vi "fpga_LP1 Process (M Class).vi"(0 "input data":fxp<+/-,32,3>, 1 "reset":bool, 2 "filter delay constant":T1, 5 "Ch":fxp<+,5,5>=6.0, 9 "input valid":bool, 12 "ready for output":bool) -> (4 "re":fxp<+/-,32,5> format="%.29g", 6 "im":fxp<+/-,32,5> format="%.29g", 10 "output valid":bool, 14 "ready for input":bool)   [LabVIEW 2013, in "NI_EP_PMU_FPGA.lvlib"]
uses:
  <vilib>/addons/Electrical Power/PMU/NI_EP_PMU_FPGA.lvlib
  <vilib>/addons/Electrical Power/PMU/FPGA/subVIs/fpga_Reporting Rate Configuration.ctl
  <vilib>/rvi/Emulation/niFpgaSctlEmulationGetInTimedLoop.vi
  <vilib>/rvi/DataTransferAndStorage/Container/Common/niFpgaContainerGetUniqueNameForEmu.vi
  <vilib>/rvi/DataTransferAndStorage/Container/Common/niFpgaContainerSetEmuInfo.vi
  <vilib>/rvi/eio/common/nirviEmuReportErrorAndStop.vi
  <vilib>/rvi/FIFO/Fifo_Resource/nirvififoEmulationSetSize.vi
  <vilib>/rvi/Emulation/niFpgaSctlEmulationFifoFullMgr.vi
  <vilib>/rvi/errors/niFpgaSetErrorForExecOnDevCompSimple.vi
  <vilib>/rvi/Memory/Memory_Emulation/nirvimemoryEmulation.vi
  <vilib>/rvi/Memory/Memory_Emulation/nirvimemoryFastEmulation.vi
  <vilib>/rvi/Memory/Memory_Emulation/niFpgaMemoryEmulationCacheClearOnFirstRun.vi
  <vilib>/rvi/Memory/Memory_Emulation/nirvimemoryEmulationManagerCache_MakeExclusive.vi
  <vilib>/rvi/Memory/Memory_Emulation/niFpgaMemoryEmulationValidateCache.vi
  <vilib>/rvi/Memory/Memory_Emulation/nirvimemoryEmulationManagerCache_ReleaseExclusive.vi
  <vilib>/rvi/Memory/Memory_Emulation/nirvimemoryEmulationManagerCache_InsertValue.vi
  <vilib>/Utility/error.llb/Clear Errors.vi
  <vilib>/rvi/Memory/Memory_Emulation/nirvimemoryEmulationManagerCache_GetValue.vi
  <vilib>/rvi/Emulation/niFpgaSctlEmulationResourceMgr.vi
  <vilib>/rvi/LocalResourceManager/LocalResourceManager.xnode
  <vilib>/rvi/DataTransferAndStorage/Container/XNode/niFpgaContainer.xnode
  <vilib>/rvi/FIFO/Fifo_Resource/nirvififoEmulationRead.vi
  <vilib>/rvi/FXPMathLib/basic elements/FxpDiscreteDelay/XNode/nifxpmath_DiscreteDelay.xnode
  <vilib>/rvi/FXPMathLib/FxpMul/XNode/nifxpmath_Multiplier.xnode
  <vilib>/rvi/FIFO/Fifo_Resource/nirvififoEmulationWrite.vi
  <vilib>/addons/Electrical Power/PQ/Resampling/NI_EP_Resample_FPGA.lvlib
  <vilib>/rvi/FXPMathLib/sim/FxpSim.dll
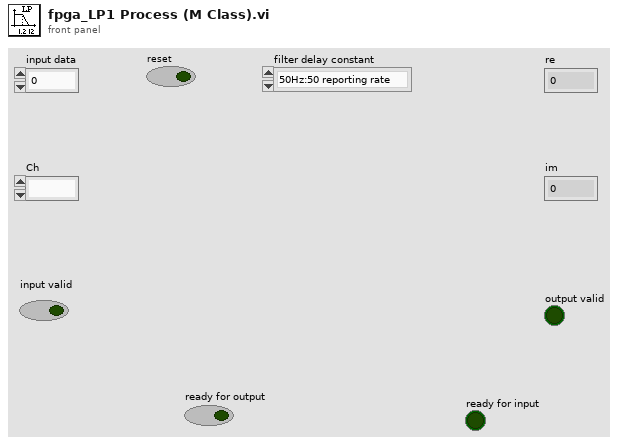
[diagram p1: front panel]
types:
  T1 = typedef "NI_EP_PMU_FPGA.lvlib/fpga_Reporting Rate Configuration.ctl" = enum16{"50Hz:50 reporting rate", "50Hz:25 reporting rate", "50Hz:10 reporting rate", "60Hz:60 reporting rate", "60Hz:30 reporting rate", "60Hz:20 reporting rate", "60Hz:15 reporting rate", "60Hz:12 reporting rate", "60Hz:10 reporting rate"}
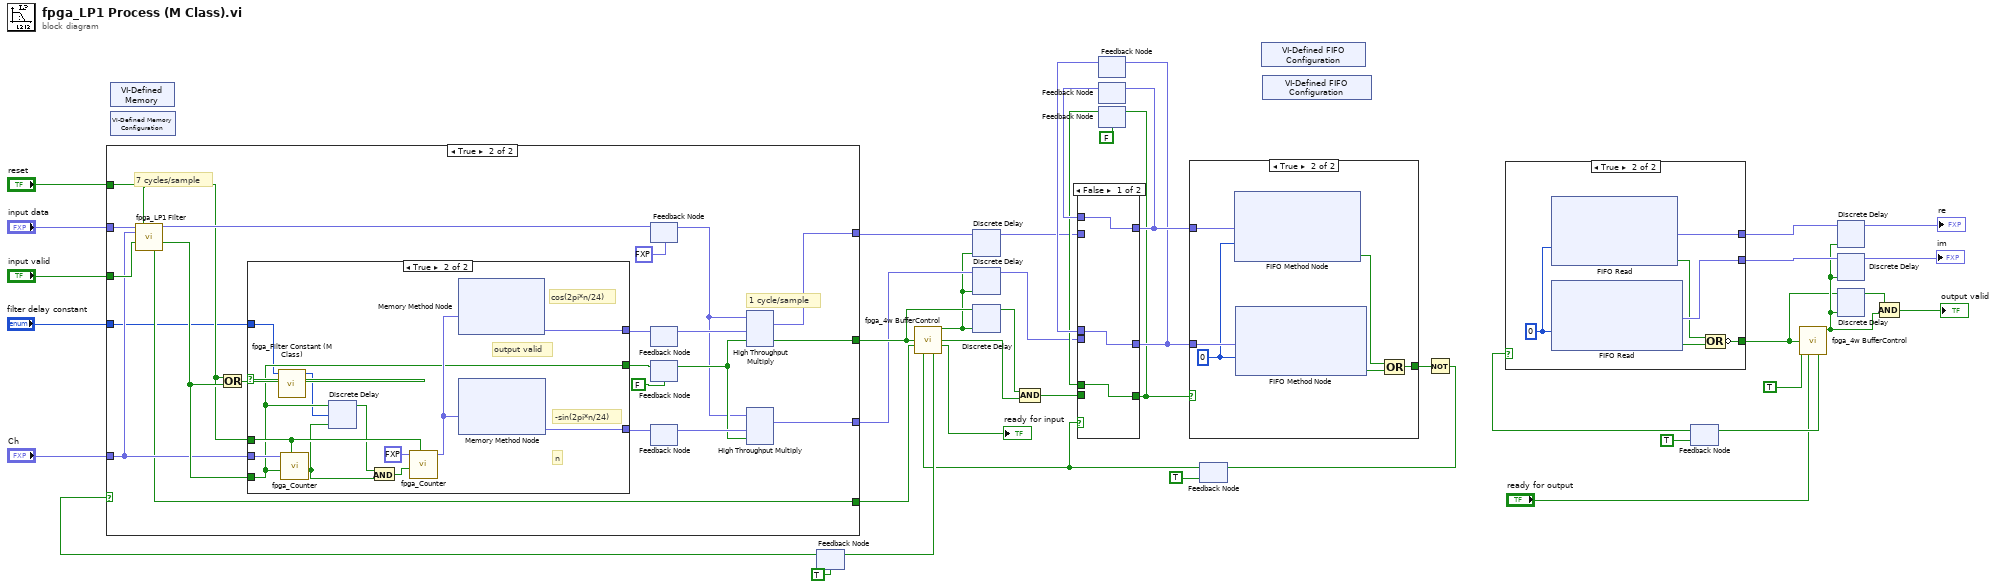
[diagram p0: block diagram]
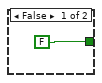
[diagram p6: hidden frame]
diagram:
  n1 = xnode "VI-Defined Memory"() -> ()  [unwired: 1 out]
  n2 = xnode "VI-Defined Memory Configuration"() -> ()  [unwired: 1 out]
  n3 = feedback #1(TRUE ("logic enable")) -> (w28:bool)
  n4 = case shown="True" w28 {
    tunnel: "input data" -> [_ w57]
    tunnel: "input valid" -> [_ w55]
    tunnel: "reset" -> [_ w52]
    tunnel: [_ w49] -> w8
    tunnel: [_ w45] -> w40
    tunnel: [_ w48] -> w7
    tunnel: [_ w47] -> w4
    tunnel: "Ch" -> [_ w46]
    tunnel: "filter delay constant" -> [_ w44]
    frame False {
    }
    frame True {
      # "1 cycle/sample"
      # "7 cycles/sample"
      n5 = call <vilib>:"fpga_LP1 Filter.vi"("input data"=w57, "reset"=w52, "#Ch"=w46, "input valid"=w55) -> ("output data"=w56:fxp<+/-,32,4>, "output valid"=w53:bool, "ready for input"=w45:bool)  [unwired: 9 in]
      n6 = Or(x=w52, y=w53) -> (x .or. y?=w54:bool)
      n7 = case shown="True" w54 {
        tunnel: [_ w76] -> w58
        tunnel: [_ w77] -> w63
        tunnel: [FALSE w69] -> w61
        tunnel: w46 -> [_ w75]
        tunnel: w53 -> [_ w69]
        tunnel: w52 -> [_ w73]
        tunnel: w44 -> [_ w66]
        frame False {
        }
        frame True {
          # "-sin(2pi*n/24)"
          # "cos(2pi*n/24)"
          # "n"
          # "output valid"
          n8 = call <vilib>:"fpga_Filter Constant (M Class).vi"("filter delay constant"=w66) -> ("LP1 delay"=w67:u8)  [unwired: 6 in, 4 out]
          n9 = call <vilib>:"fpga_Counter.vi"("reset"=w73, "Input Valid?"=w69, "upper limit"=w75) -> ("Multichannel Valid?"=w70:bool)  [unwired: 7 in, 1 out]
          n10 = xnode ("Discrete Delay")("D"=w69, "n-1[0..15]"=w67, "enable"=w70) -> ("Q"=w68:bool)
          n11 = And(x=w68, y=w70) -> (x .and. y?=w74:bool)
          n12 = call <vilib>:"fpga_Counter.vi"("reset"=w73, "Input Valid?"=w74, "upper limit"=fxp<+,5,5> 24.0 ("#ch")) -> ("count"=w72:fxp<+,5,5>)  [unwired: 7 in, 1 out]
          n13 = xnode ("Memory Method Node")("Address"=w72) -> ("Data"=w76:fxp<+/-,32,2>)  [unwired: 1 in, 1 out]
          n14 = xnode ("Memory Method Node")("Address"=w72) -> ("Data"=w77:fxp<+/-,32,2>)  [unwired: 1 in, 1 out]
        }
      }
      n15 = feedback #2(fxp<+/-,32,4> 0.0 ("output data")) -> (w50:fxp<+/-,32,4>)
      n16 = feedback-in #2(w56) -> ()
      n17 = feedback #3() -> (w51:fxp<+/-,32,2>)  [unwired: 1 in]
      n18 = feedback-in #3(w58) -> ()
      n19 = feedback #4(FALSE) -> (w60:bool)
      n20 = feedback-in #4(w61) -> ()
      n21 = feedback #5() -> (w62:fxp<+/-,32,2>)  [unwired: 1 in]
      n22 = feedback-in #5(w63) -> ()
      n23 = xnode ("High Throughput Multiply")("x"=w50, "y"=w51, "input valid"=w60) -> ("x*y"=w48:fxp<+/-,32,5>, "output valid"=w49:bool)  [unwired: 1 in, 1 out]
      n24 = xnode ("High Throughput Multiply")("x"=w50, "y"=w62, "input valid"=w60) -> ("x*y"=w47:fxp<+/-,32,5>)  [unwired: 1 in, 2 out]
    }
  }
  n25 = feedback #6() -> (w38:fxp<+/-,32,5>)  [unwired: 1 in]
  n26 = feedback #7() -> (w39:fxp<+/-,32,5>)  [unwired: 1 in]
  n27 = feedback #8(FALSE) -> (w34:bool)
  n28 = feedback #9(TRUE) -> (w25:bool)
  n29 = call <vilib>:"fpga_4w BufferControl.vi"("DR"=w8, "RFI"=w40, "RFO"=w25) -> ("buff enable"=w3:bool, "output valid"=w31:bool, "ready for input"=→"ready for input":bool, "logic enable"=w29:bool)  [unwired: 9 in]
  n30 = feedback-in #1(w29) -> ()
  n31 = xnode ("Discrete Delay")("D"=w7, "enable"=w3) -> ("Q"=w6:fxp<+/-,32,5>)
  n32 = xnode ("Discrete Delay")("D"=w4, "enable"=w3) -> ("Q"=w2:fxp<+/-,32,5>)
  n33 = xnode ("Discrete Delay")("D"=w8, "enable"=w3) -> ("Q"=w5:bool)
  n34 = Compound Arithmetic op=AND(w5, w31) -> (w32:bool)
  n35 = case shown="False" w25 {
    tunnel: w6 -> [_ w83]
    tunnel: w32 -> [_ w81]
    tunnel: w2 -> [_ w82]
    tunnel: [w80 w83] -> w37
    tunnel: w39 -> [w80 _]
    tunnel: [w79 w82] -> w30
    tunnel: w38 -> [w79 _]
    tunnel: [w78 w81] -> w13
    tunnel: w34 -> [w78 _]
    frame False {
    }
    frame True {
    }
  }
  n36 = feedback-in #6(w30) -> ()
  n37 = feedback-in #7(w37) -> ()
  n38 = feedback-in #8(w13) -> ()
  n39 = case shown="True" w13 {
    tunnel: w37 -> [_ w89]
    tunnel: w30 -> [_ w88]
    tunnel: [_ w84] -> w36
    frame False {
    }
    frame True {
      w87 = 0 ("Timeout")
      n40 = xnode ("FIFO Method Node")("Element"=w89, "Timeout"=w87) -> ("Timed Out?"=w85:bool)  [unwired: 1 in, 1 out]
      n41 = xnode ("FIFO Method Node")("Element"=w88, "Timeout"=w87) -> ("Timed Out?"=w86:bool)  [unwired: 1 in, 1 out]
      n42 = Compound Arithmetic op=OR(w85, w86) -> (w84:bool)
    }
  }
  n43 = xnode "VI-Defined FIFO Configuration"() -> ()  [unwired: 1 out]
  n44 = xnode "VI-Defined FIFO Configuration"() -> ()  [unwired: 1 out]
  n45 = Not(x=w36) -> (.not. x?=w9:bool)
  n46 = feedback-in #9(w9) -> ()
  n47 = feedback #10(TRUE ("logic enable")) -> (w22:bool)
  n48 = case shown="True" w22 {
    tunnel: [_ w95] -> w12
    tunnel: [_ w94] -> w19
    tunnel: [_ w92] -> w11
    frame False {
    }
    frame True {
      w93 = 0 ("Timeout")
      n49 = xnode ("FIFO Read")("Timeout"=w93) -> ("Element"=w92:fxp<+/-,32,5>, "Timed Out?"=w91:bool)  [unwired: 1 in, 1 out]
      n50 = xnode ("FIFO Read")("Timeout"=w93) -> ("Element"=w94:fxp<+/-,32,5>, "Timed Out?"=w90:bool)  [unwired: 1 in, 1 out]
      n51 = Compound Arithmetic op=OR(w91, w90) -> (invert w95:bool)
    }
  }
  n52 = call <vilib>:"fpga_4w BufferControl.vi"("DR"=w12, "RFI"=TRUE, "RFO"="ready for output") -> ("buff enable"=w14:bool, "logic enable"=w23:bool)  [unwired: 9 in, 2 out]
  n53 = feedback-in #10(w23) -> ()
  n54 = xnode ("Discrete Delay")("D"=w11, "enable"=w14) -> ("Q"=→"re":fxp<+/-,32,5>)
  n55 = xnode ("Discrete Delay")("D"=w19, "enable"=w14) -> ("Q"=→"im":fxp<+/-,32,5>)
  n56 = xnode ("Discrete Delay")("D"=w12, "enable"=w14) -> ("Q"=w21:bool)
  n57 = Compound Arithmetic op=AND(w21, w14) -> (→"output valid":bool)
